vi "Send Shutdown.vi"(8 "error in (no error)":errorcluster, 11 "Dispatcher Interface in":refnum<class "Dispatcher Interface.lvclass">) -> (0 "error out":errorcluster, 3 "Dispatcher Interface out":refnum<class "Dispatcher Interface.lvclass">)   [LabVIEW 2021, in "DSF Core.lvlib" / "Dispatcher Interface.lvclass"]
uses:
  Dispatcher Interface.lvclass
  C:/dev/git/custom-devices/niveristand-data-sharing-framework-custom-device/Source/Core/Classes/Interface/Interface.lvclass
  Command.ctl
  Command Data.ctl
  Parameters.ctl
  Response.ctl
  Write Dispatcher Command.vi
  Read Dispatcher Response.vi
  Invalid Response.vi
  Interface.lvclass
  Read Dispatcher Error.vi
  C:/dev/git/custom-devices/niveristand-data-sharing-framework-custom-device/Source/Core/Classes/Interface/Dispatcher/Dispatcher Interface.lvclass
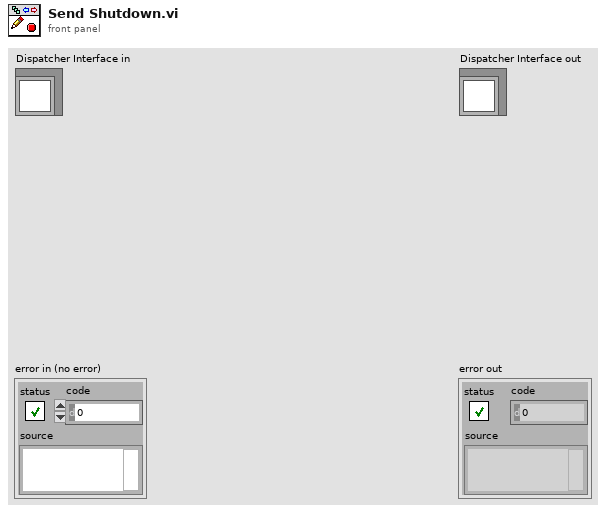
[diagram p1: front panel]
types:
  T1 = typedef "DSF Core.lvlib/Dispatcher Interface.lvclass/Command.ctl" = enum8{"Idle", "Start", "Rx", "Tx", "Set Inline Buffer", "Shutdown", "Error"}
  T2 = typedef "DSF Core.lvlib/Dispatcher Interface.lvclass/Command Data.ctl" = cluster{"Command":T1, "Parameters":T3}
  T3 = typedef "DSF Core.lvlib/Dispatcher Interface.lvclass/Parameters.ctl" = cluster{"arg1":u64, "arg2":u64}
  T4 = typedef "DSF Core.lvlib/Dispatcher Interface.lvclass/Response Data.ctl" = cluster{"Response":T5, "Parameters":T3}
  T5 = typedef "DSF Core.lvlib/Dispatcher Interface.lvclass/Response.ctl" = enum8{"General Ack", "Error", "Shutting Down"}
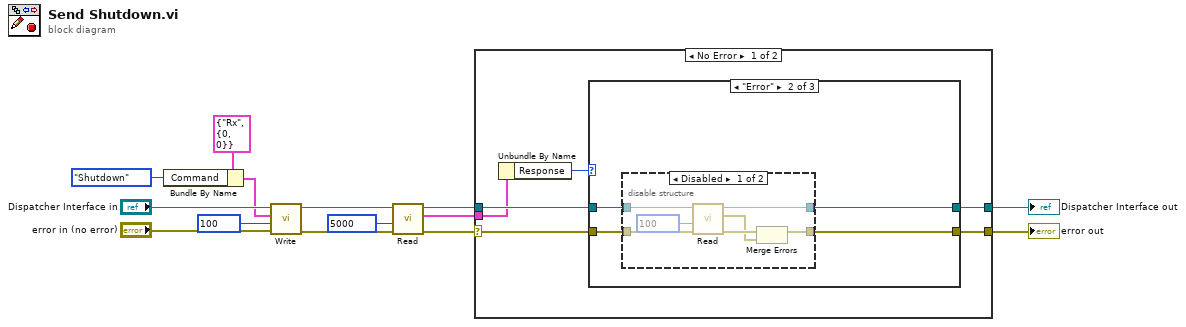
[diagram p0: block diagram]
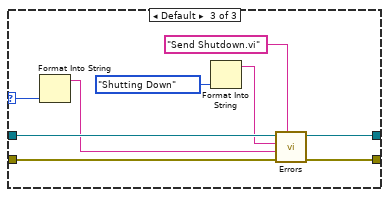
[diagram p4: hidden frame]
diagram:
  n1 = Bundle By Name(cluster=T2 {"Command"=enum."Rx", "Parameters"={"arg1"=0, "arg2"=0}} ("command"), "Command"=Command."Shutdown") -> (w10:T2)
  n2 = call-poly "Write.vi"("error in (no error)"="error in (no error)", "timeout in ms (0)"=100, "command"=w10, "Dispatcher Interface in"="Dispatcher Interface in") -> ("error out"=w6:errorcluster, "Dispatcher Interface out"=w7:refnum<class "Dispatcher Interface.lvclass">)  [unwired: 6 in]
  n3 = call-poly "Read.vi"("error in (no error)"=w6, "timeout in ms (0)"=5000, "Dispatcher Interface in"=w7) -> ("error out"=w4:errorcluster, "response"=w1:T4, "Dispatcher Interface out"=w5:refnum<class "Dispatcher Interface.lvclass">)  [unwired: 5 in, 1 out]
  n4 = case shown="No Error" w4 {
    selector: w4 -> [w15 w45]
    tunnel: [w19 w45] -> w2
    tunnel: w5 -> [w18 w46]
    tunnel: [w17 w46] -> w3
    tunnel: w1 -> [w16 _]
    frame No Error {
      n5 = Unbundle By Name(w16) -> ("Response"=w20:T5)
      n6 = case shown="\"Error\"" w20 {
        selector: w20 -> [_ _ w40]
        tunnel: w15 -> [w21 w25 w43]
        tunnel: [w21 w23 w41] -> w19
        tunnel: w18 -> [w22 w26 w44]
        tunnel: [w22 w24 w42] -> w17
        frame "Shutting Down" {
          # "Valid response."
        }
        frame "Error" {
          n7 = disable-structure shown="Disabled" {
            disable-tunnel: w26 -> [w33 w35]
            disable-tunnel: w25 -> [w32 w34]
            disable-tunnel: [w30 w35] -> w24
            disable-tunnel: [w28 w34] -> w23
            frame Disabled {
              n8 = call-poly "Read.vi"("error in (no error)"=w32, "timeout in ms (0)"=100, "Dispatcher Interface in"=w33) -> ("error out"=w29:errorcluster, "error"=w27:errorcluster, "Dispatcher Interface out"=w30:refnum<class "Dispatcher Interface.lvclass">)  [unwired: 6 in]
              n9 = Merge Errors(w29, w27) -> (w28:errorcluster)
            }
            frame Enabled {
            }
          }
        }
        frame Default {
          n10 = Format Into String(w40) -> (resulting string=w39:string)  [unwired: 3 in, 1 out]
          n11 = Format Into String(Response."Shutting Down" ("Response")) -> (resulting string=w38:string)  [unwired: 3 in, 1 out]
          n12 = call-poly "Errors.vi"("error source vi name"="Send Shutdown.vi", "error in (no error)"=w43, "actual response"=w39, "expected response"=w38, "Interface in"=w44) -> ("error out"=w41:errorcluster, "Interface out"=w42:refnum<class "Dispatcher Interface.lvclass">)  [unwired: 5 in]
        }
      }
    }
    frame Error {
      # "Incoming error. Pass through."
    }
  }
  "error out" <- w2
  "Dispatcher Interface out" <- w3
